vi "fade.vi"(6 "Iteration_Num":dbl, 7 "Color Array":u32[](array[colorbox]), 9 "Length":dbl, 10 "fade constant":dbl, 11 "Wait_Constant":dbl) -> (3 "Output_Array":u32[](array[colorbox]))   [LabVIEW 2020]
panel:
  in  "Color_Start":u32(colorbox)
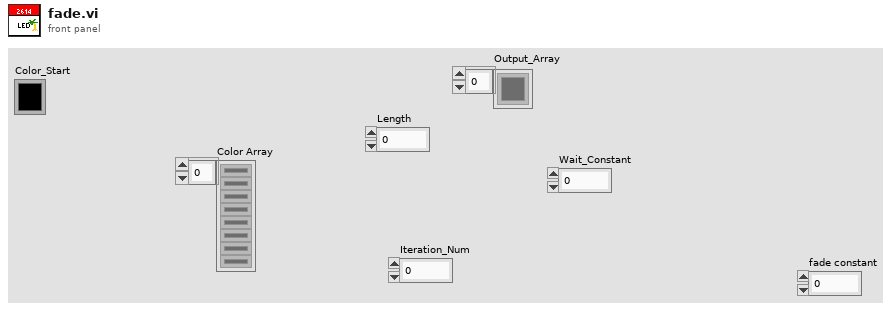
[diagram p1: front panel]
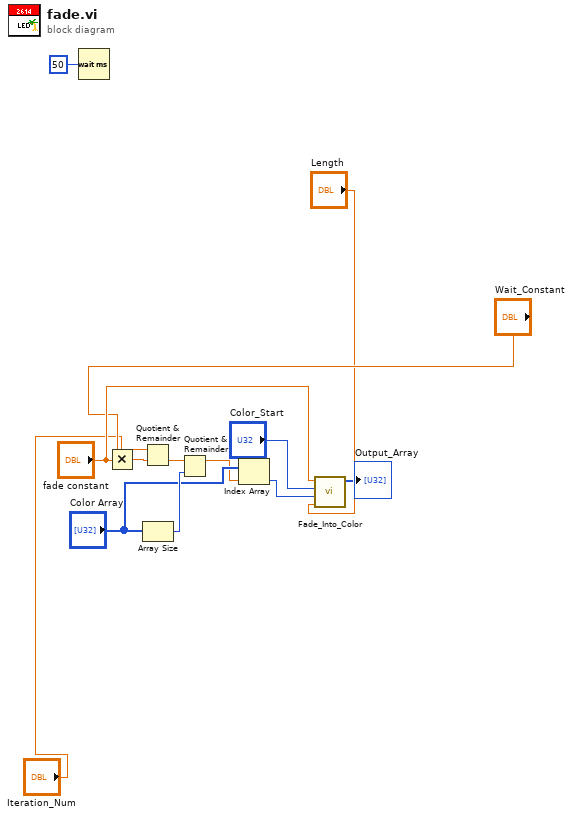
[diagram p0: block diagram]
diagram:
  n1 = Wait (ms)(milliseconds to wait=u32 50) -> ()  [unwired: 1 out]
  n2 = Multiply(x="fade constant", y="Wait_Constant") -> (x*y=w6:dbl)
  n3 = Quotient & Remainder(x="Iteration_Num", y=w6) -> (floor(x/y)=w12:dbl)  [unwired: 1 out]
  n4 = Array Size(array="Color Array") -> (size(s)=w11:i32)
  n5 = Quotient & Remainder(x=w12, y=w11) -> (x-y*floor(x/y)=w9:dbl)  [unwired: 1 out]
  n6 = Index Array(array="Color Array", index=w9) -> (element=w8:u32)
  n7 = call "Fade_Into_Color.vi"("Length"="Length", "Color_Goal"=w8, "Color_Start"="Color_Start", "fade constant"="fade constant") -> ("Output_Array"=→"Output_Array":u32[])  [unwired: 7 in]
